vi "Read Drive Operation.vi"(8 "Command Info":T4) -> (0 "Command Info":T4, 1 "SubSystem Data":T1={"Operation"=enum."Reserve", "Left Setpoint"=0.0, "Right Setpoint"=0.0, "Duration"=0.0, "RobotNeededPathData"={"Path"=[], "MaxVel"=0.0, "MaxAccel"=0.0, "Backwards?"=FALSE, "PointSpacing"=0.0, "LookaheadDist"=0.0, "Speed/Curve"=1.8, "SlowDistanceAtEnd"=12.0, "SlowSpeed"=15.0, "MaxDeAccel"=0.0}, "Angle"=0.0, "Distance"=0.0, "UseVision"=FALSE} {"RobotNeededPathData"."SlowSpeed" format="%#_13g"; "RobotNeededPathData"."SlowDistanceAtEnd" format="%#_13g"; "RobotNeededPathData"."Speed/Curve" format="%#_13g"}, 2 "Command Timing":cluster{"Start Time (ms)":u32, "Iterations":i32})   [LabVIEW 2018]
doc: "Returns the details about the currently executing command."
uses:
  <vilib>/Rock Robotics/WPI/Framework/Command Status Info.ctl
  <vilib>/Rock Robotics/WPI/Framework/Completion Status.ctl
  <vilib>/Rock Robotics/WPI/Framework/Completion Notifier.ctl
  Implementation/Drive Setpoints.ctl
  Implementation/Drive Operations.ctl
  Dawgma Programming Library/Controls/PurePursuit/RobotNeededPathData.ctl
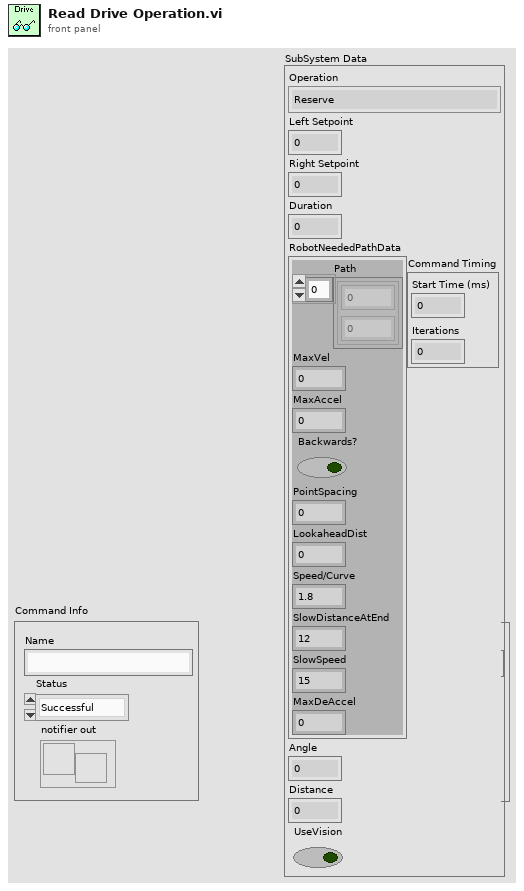
[diagram p1: front panel]
types:
  T1 = typedef "Drive Setpoints.ctl" = cluster{"Operation":T2, "Left Setpoint":dbl, "Right Setpoint":dbl, "Duration":dbl, "RobotNeededPathData":T3, "Angle":dbl, "Distance":dbl, "UseVision":bool}
  T2 = typedef "Drive Operations.ctl" = enum16{"Reserve", "Read Current", "Immediate", "Drive for Time", "Drive for Distance", "Drive Path", "Turn to Angle"}
  T3 = typedef "RobotNeededPathData.ctl" = cluster{"Path":cluster{dbl, dbl}[], "MaxVel":dbl, "MaxAccel":dbl, "Backwards?":bool, "PointSpacing":dbl, "LookaheadDist":dbl, "Speed/Curve":dbl, "SlowDistanceAtEnd":dbl, "SlowSpeed":dbl, "MaxDeAccel":dbl}
  T4 = typedef "Command Status Info.ctl" = cluster{"Name":string, "Status":T5, "notifier out":T6}
  T5 = typedef "Completion Status.ctl" = enum16{"Successful", "Aborted", "Incomplete"}
  T6 = typedef "Completion Notifier.ctl" = refnum<notifier>
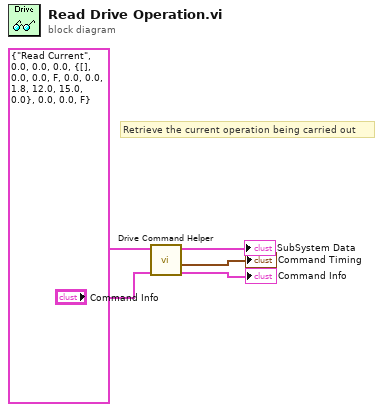
[diagram p0: block diagram]
diagram:
  # "Retrieve the current operation being carried out"
  n1 = call "Drive Command Helper.vi"("Command Info In"="Command Info", "SubSystem Data"=T1 {"Operation"=enum."Read Current", "Left Setpoint"=0.0, "Right Setpoint"=0.0, "Duration"=0.0, "RobotNeededPathData"={"Path"=[], "MaxVel"=0.0, "MaxAccel"=0.0, "Backwards?"=FALSE, "PointSpacing"=0.0, "LookaheadDist"=0.0, "Speed/Curve"=1.8, "SlowDistanceAtEnd"=12.0, "SlowSpeed"=15.0, "MaxDeAccel"=0.0}, "Angle"=0.0, "Distance"=0.0, "UseVision"=FALSE}) -> ("Command Info Out"=→"Command Info":T4, "Command Timing"=→"Command Timing":cluster{"Start Time (ms)":u32, "Iterations":i32}, "SubSystem Data"=→"SubSystem Data":T1)  [unwired: 7 in]
